vi "Build Datagram.vi"(4 "destination address":u32, 5 "transfer id":i32, 6 "destination port":u16, 7 "transfer group id":i32, 8 "error in (no error)":errorcluster, 10 "transfer data":string, 11 "UDP Transceiver in":refnum<class "UDP Transceiver.lvclass">) -> (0 "error out":errorcluster, 2 "datagram":string, 3 "UDP Transceiver out":refnum<class "UDP Transceiver.lvclass">)   [LabVIEW 2020, in "UDP.lvlib" / "UDP Transceiver.lvclass"]
uses:
  UDP Transceiver.lvclass
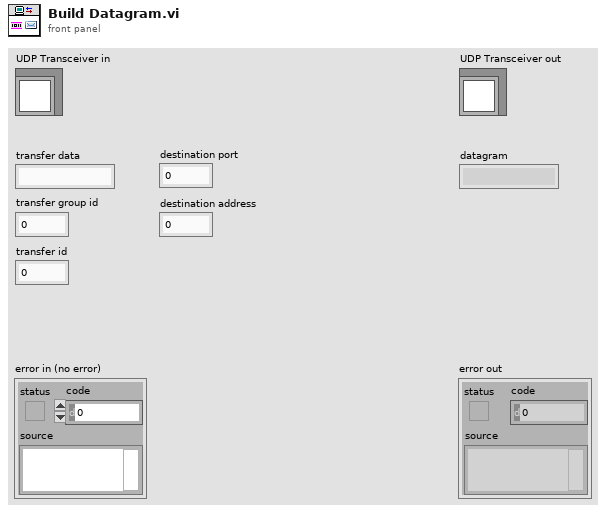
[diagram p1: front panel]
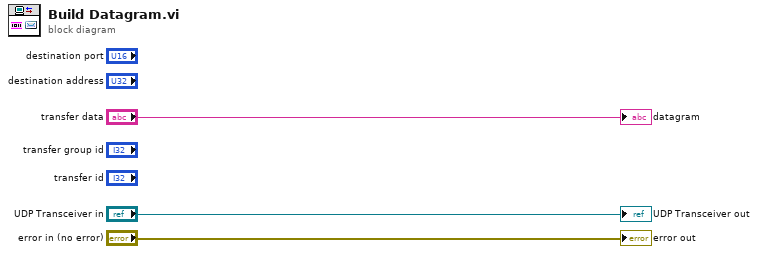
[diagram p0: block diagram]
diagram:
  "error out" <- "error in (no error)"
  "UDP Transceiver out" <- "UDP Transceiver in"
  "datagram" <- "transfer data"
